vi "pattern_matching.vi"() -> ()   [LabVIEW 2014]
uses:
  <vilib>/userdefined/High Color/IMAQdx.ctl
  <vilib>/vision/Avi1.llb/AviRefnum.ctl
  <vilib>/vision/driver/NI_Vision_Acquisition_Software.lvlib
  <vilib>/vision/NI_Vision_Development_Module.lvlib
  <resource>/objmgr/imaqdx.rc
panel:
  in  "Länge der Spur":i32=50
  in  "Frames Per Second":u32=20
  in  "BayerPattern":u32(ring)=5 items=["None", "GB", "GR", "BG", "RG", "Use Hardware Value"]
  out "ValueString":string
  out "ValueBool":bool
  out "IPAddress":string
  in  "y":i32
  in  "x":i32
  in  "Pattern2 Farbe":u32(colorbox)=16711680
  in  "pattern3":bool
  in  "y 3":i32
  in  "x 3":i32
  out "Pattern 5":T1(plugin-control)
  in  "Pattern5 Farbe":u32(colorbox)=16711680
  in  "pattern5":bool
  in  "y 5":i32
  in  "x 5":i32
  in  "Pattern4 Farbe":u32(colorbox)=16711680
  in  "pattern4":bool
  in  "y 4":i32
  in  "x 4":i32
  out "Pattern 4":T1(plugin-control)
  in  "Template File Path (Pattern Matching 4":path=path "C:/Users/Kroll/Desktop/Test_04012016/Pattern/templet_invertiert_2.png"
  in  "Template File Path (Pattern Matching 5":path=path "C:/Users/Kroll/Desktop/Test_04012016/Pattern/TEST_PAINT.png"
  in  "Pattern2 Farbe":u32(colorbox)=16711680
  in  "pattern2":bool
  out "Pattern 3":T1(plugin-control)
  in  "Template File Path (Pattern Matching 3":path=path "C:/Users/Kroll/Desktop/Test_04012016/Pattern/pattern3.png"
  out "Pattern1":T1(plugin-control)
  out "Pattern 2":T1(plugin-control)
  in  "Pattern1 Farbe":u32(colorbox)=16711680
  in  "pattern1":bool
  out "Acquired Frames/s":dbl
  in  "Länge des Pfeils":sgl=80.0
  in  "Aufnahme Starten":bool
  out "Selected Path":path
  in  "Max Data Size":u32=10000
  in  "y 2":i32
  in  "x 2":i32
  out "Processed Frames/s":dbl
  in  "Template File Path (Pattern Matching 2":path=path "C:/Users/Kroll/Desktop/Test_04012016/Pattern/pattern_test_1412.png"
  in  "millisecond multiple":u32
  in  "Mittelpunktgröße":sgl
  out "date/time string":string
  in  "file path (dialog if empty)":path=path "I:/123.txt"
  in  "Template File Path (Pattern Matching 1)":path=path "C:/Users/Kroll/Desktop/Test_04012016/Pattern/pattern_1412.png"
  in  "Parameters Pattern":T2={"Number of Matches Requested"=1, "Minimum Match Score"=800.0, "Angle Ranges"=[{"Start Angle"=-180.0, "End Angle"=180.0}, {"Start Angle"=0.0, "End Angle"=360.0}]}
  in  "Programm anhalten":bool
  out "Threshold Image 2":T1(plugin-control)
  out "Image 2":T1(plugin-control)
  # "Speicherort der Log Datei"
  # "Program Delay einstellen"
  # "Zum Rauszoomen Shift benutzen ->"
  # "Aufnahme"
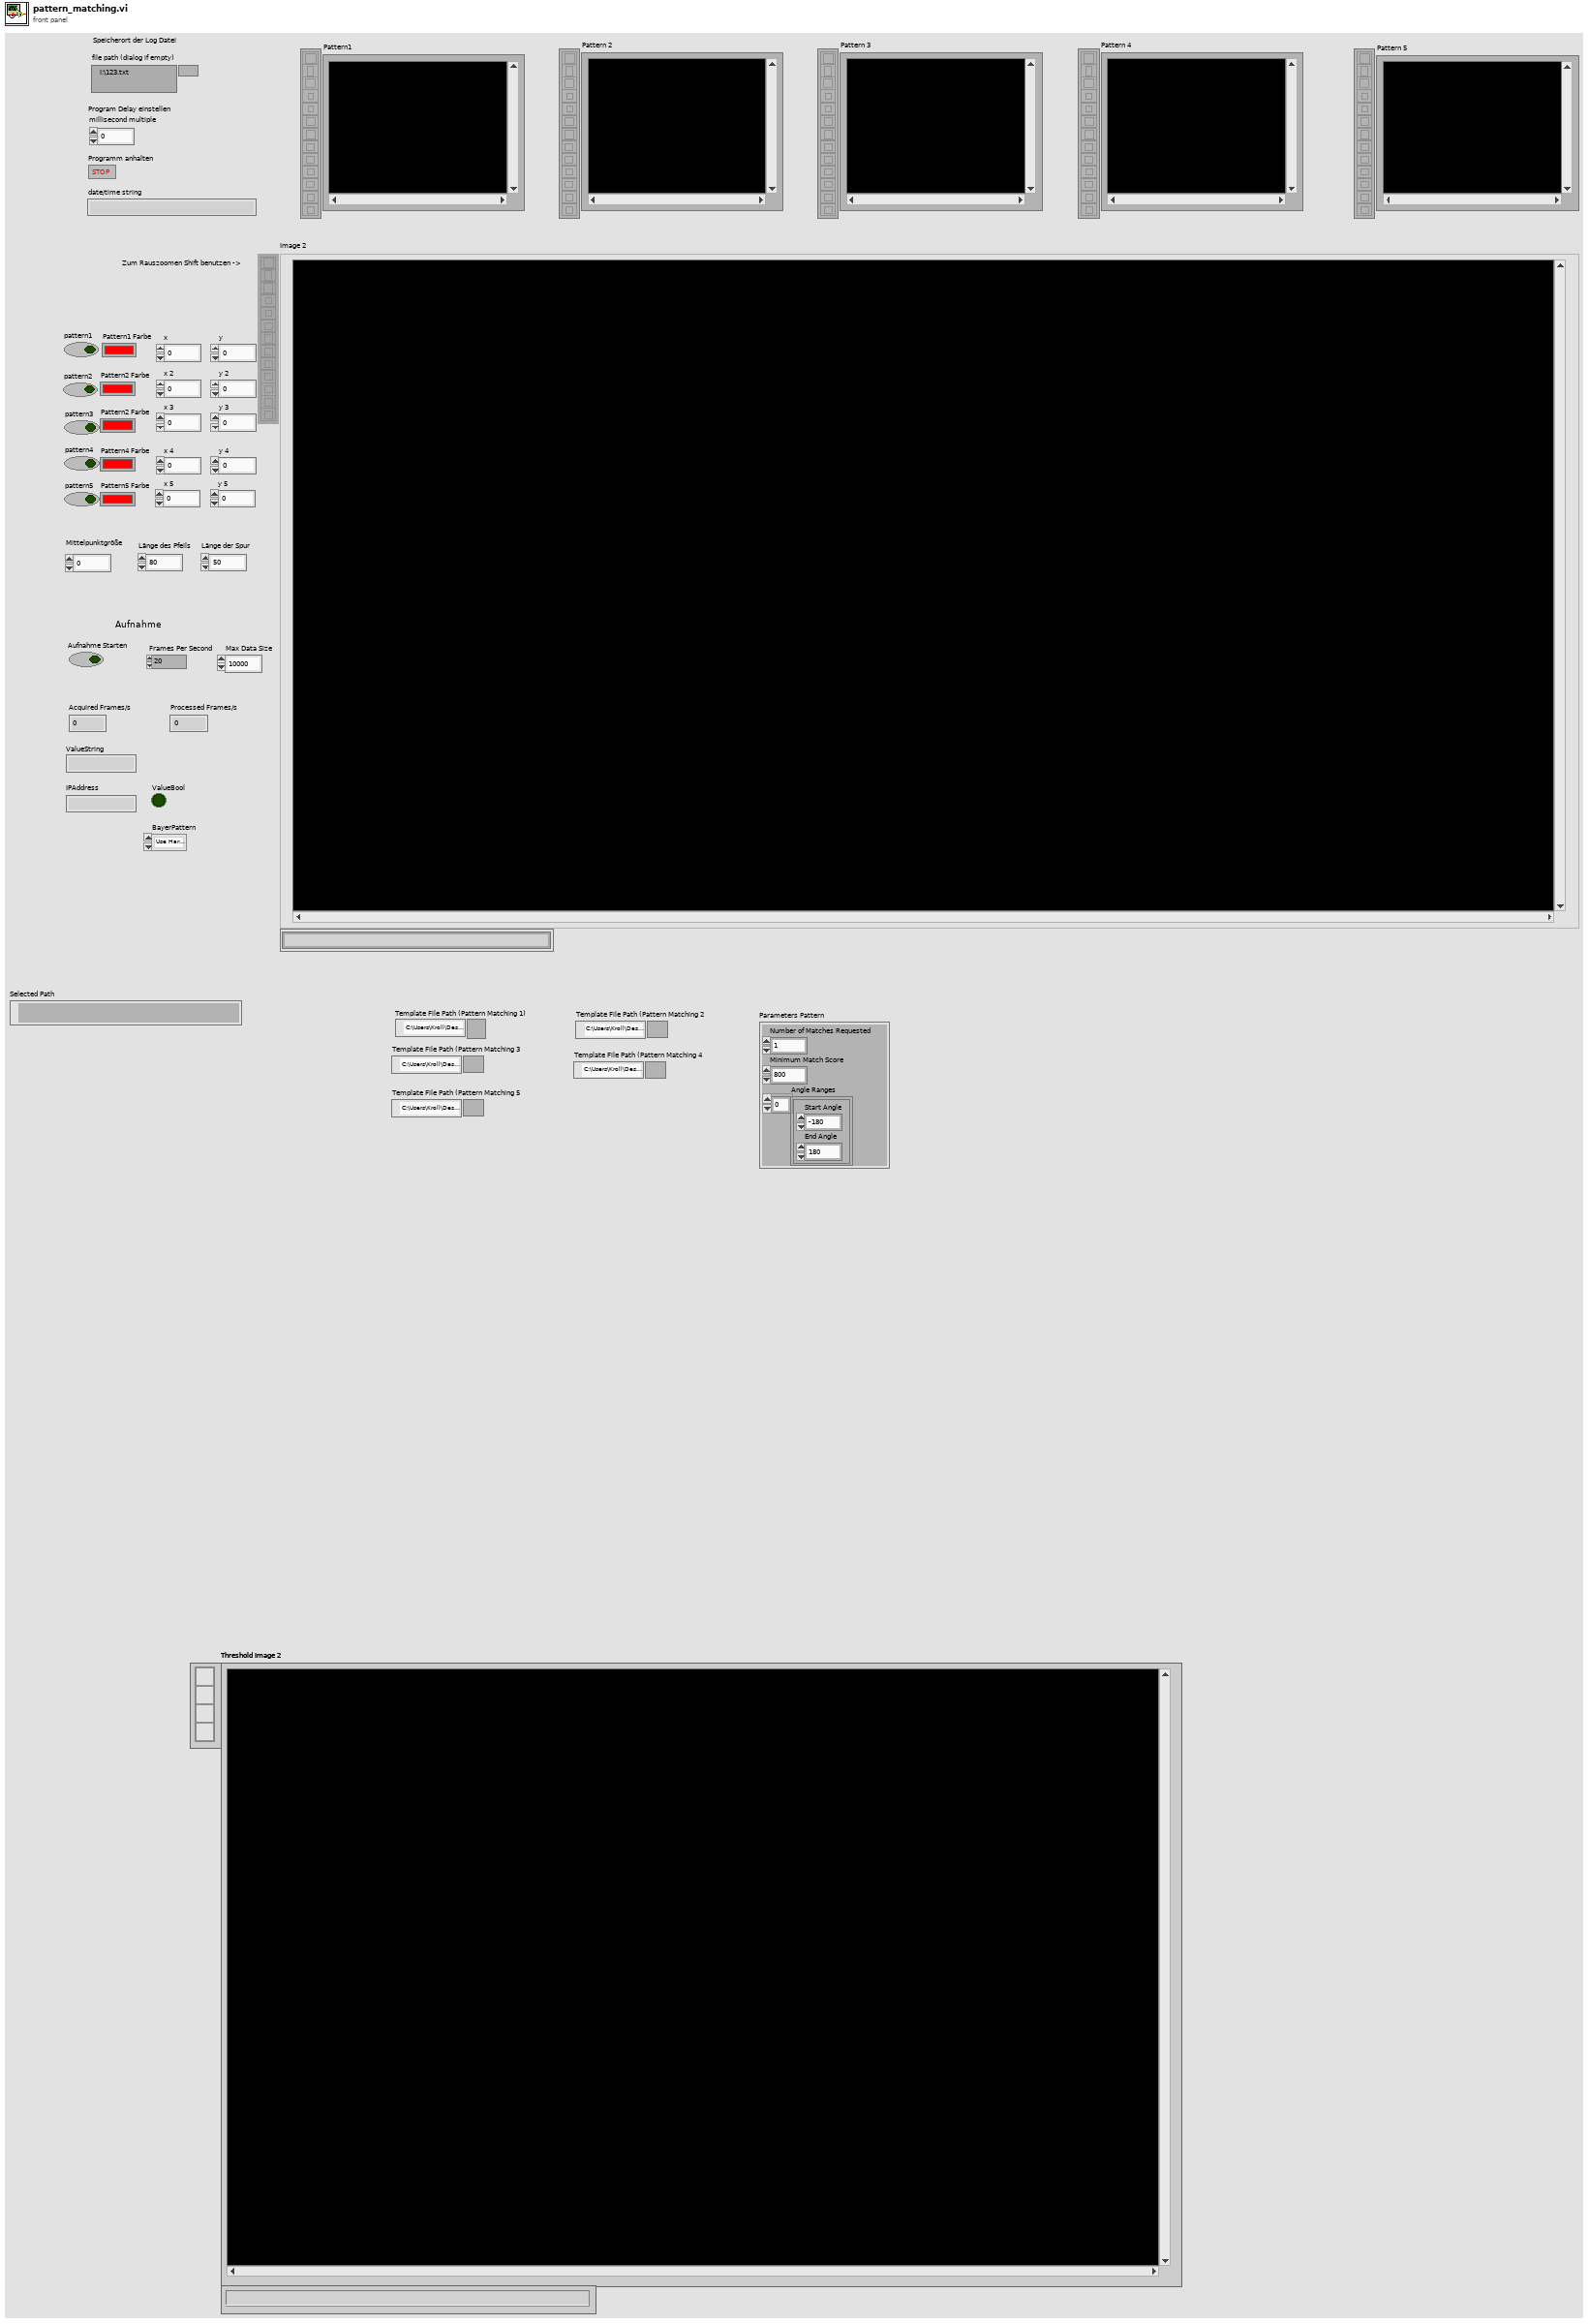
[diagram p1: front panel]
types:
  T1 = typedef "IMAQ Image.ctl" = refnum<image>
  T2 = cluster{"Number of Matches Requested":i32, "Minimum Match Score":sgl, "Angle Ranges":cluster{"Start Angle":sgl, "End Angle":sgl}[]}
  T3 = typedef "IMAQdx.ctl" = refnum<k21>
  T4 = typedef "Image Type" = u32
  T5 = enum16{"open", "replace", "create", "open or create", "replace or create", "replace or create with confirmation"}
  T6 = typedef "AviRefnum.ctl" = refnum<k1>
  T7 = enum32{"existing file", "new file", "new or existing file", "existing dir", "new dir", "new or existing dir", "existing file (use LLBs)", "new file (use LLBs)", "new or existing file (use LLBs)", "new or existing file or directory (use LLBs)"}
  T8 = cluster{"Position":cluster{"x":sgl, "y":sgl}, "Angle":sgl, "Scale":sgl, "Score":sgl, "Bounding Box":cluster{"x":sgl, "y":sgl}[]}[]
  T9 = typedef "ROI Descriptor" = cluster{"Global Rectangle":i32[], "Contours":cluster{"ID":enum32{"External", "Internal"}, "Type":u32, "Coordinates":i32[]}[]}
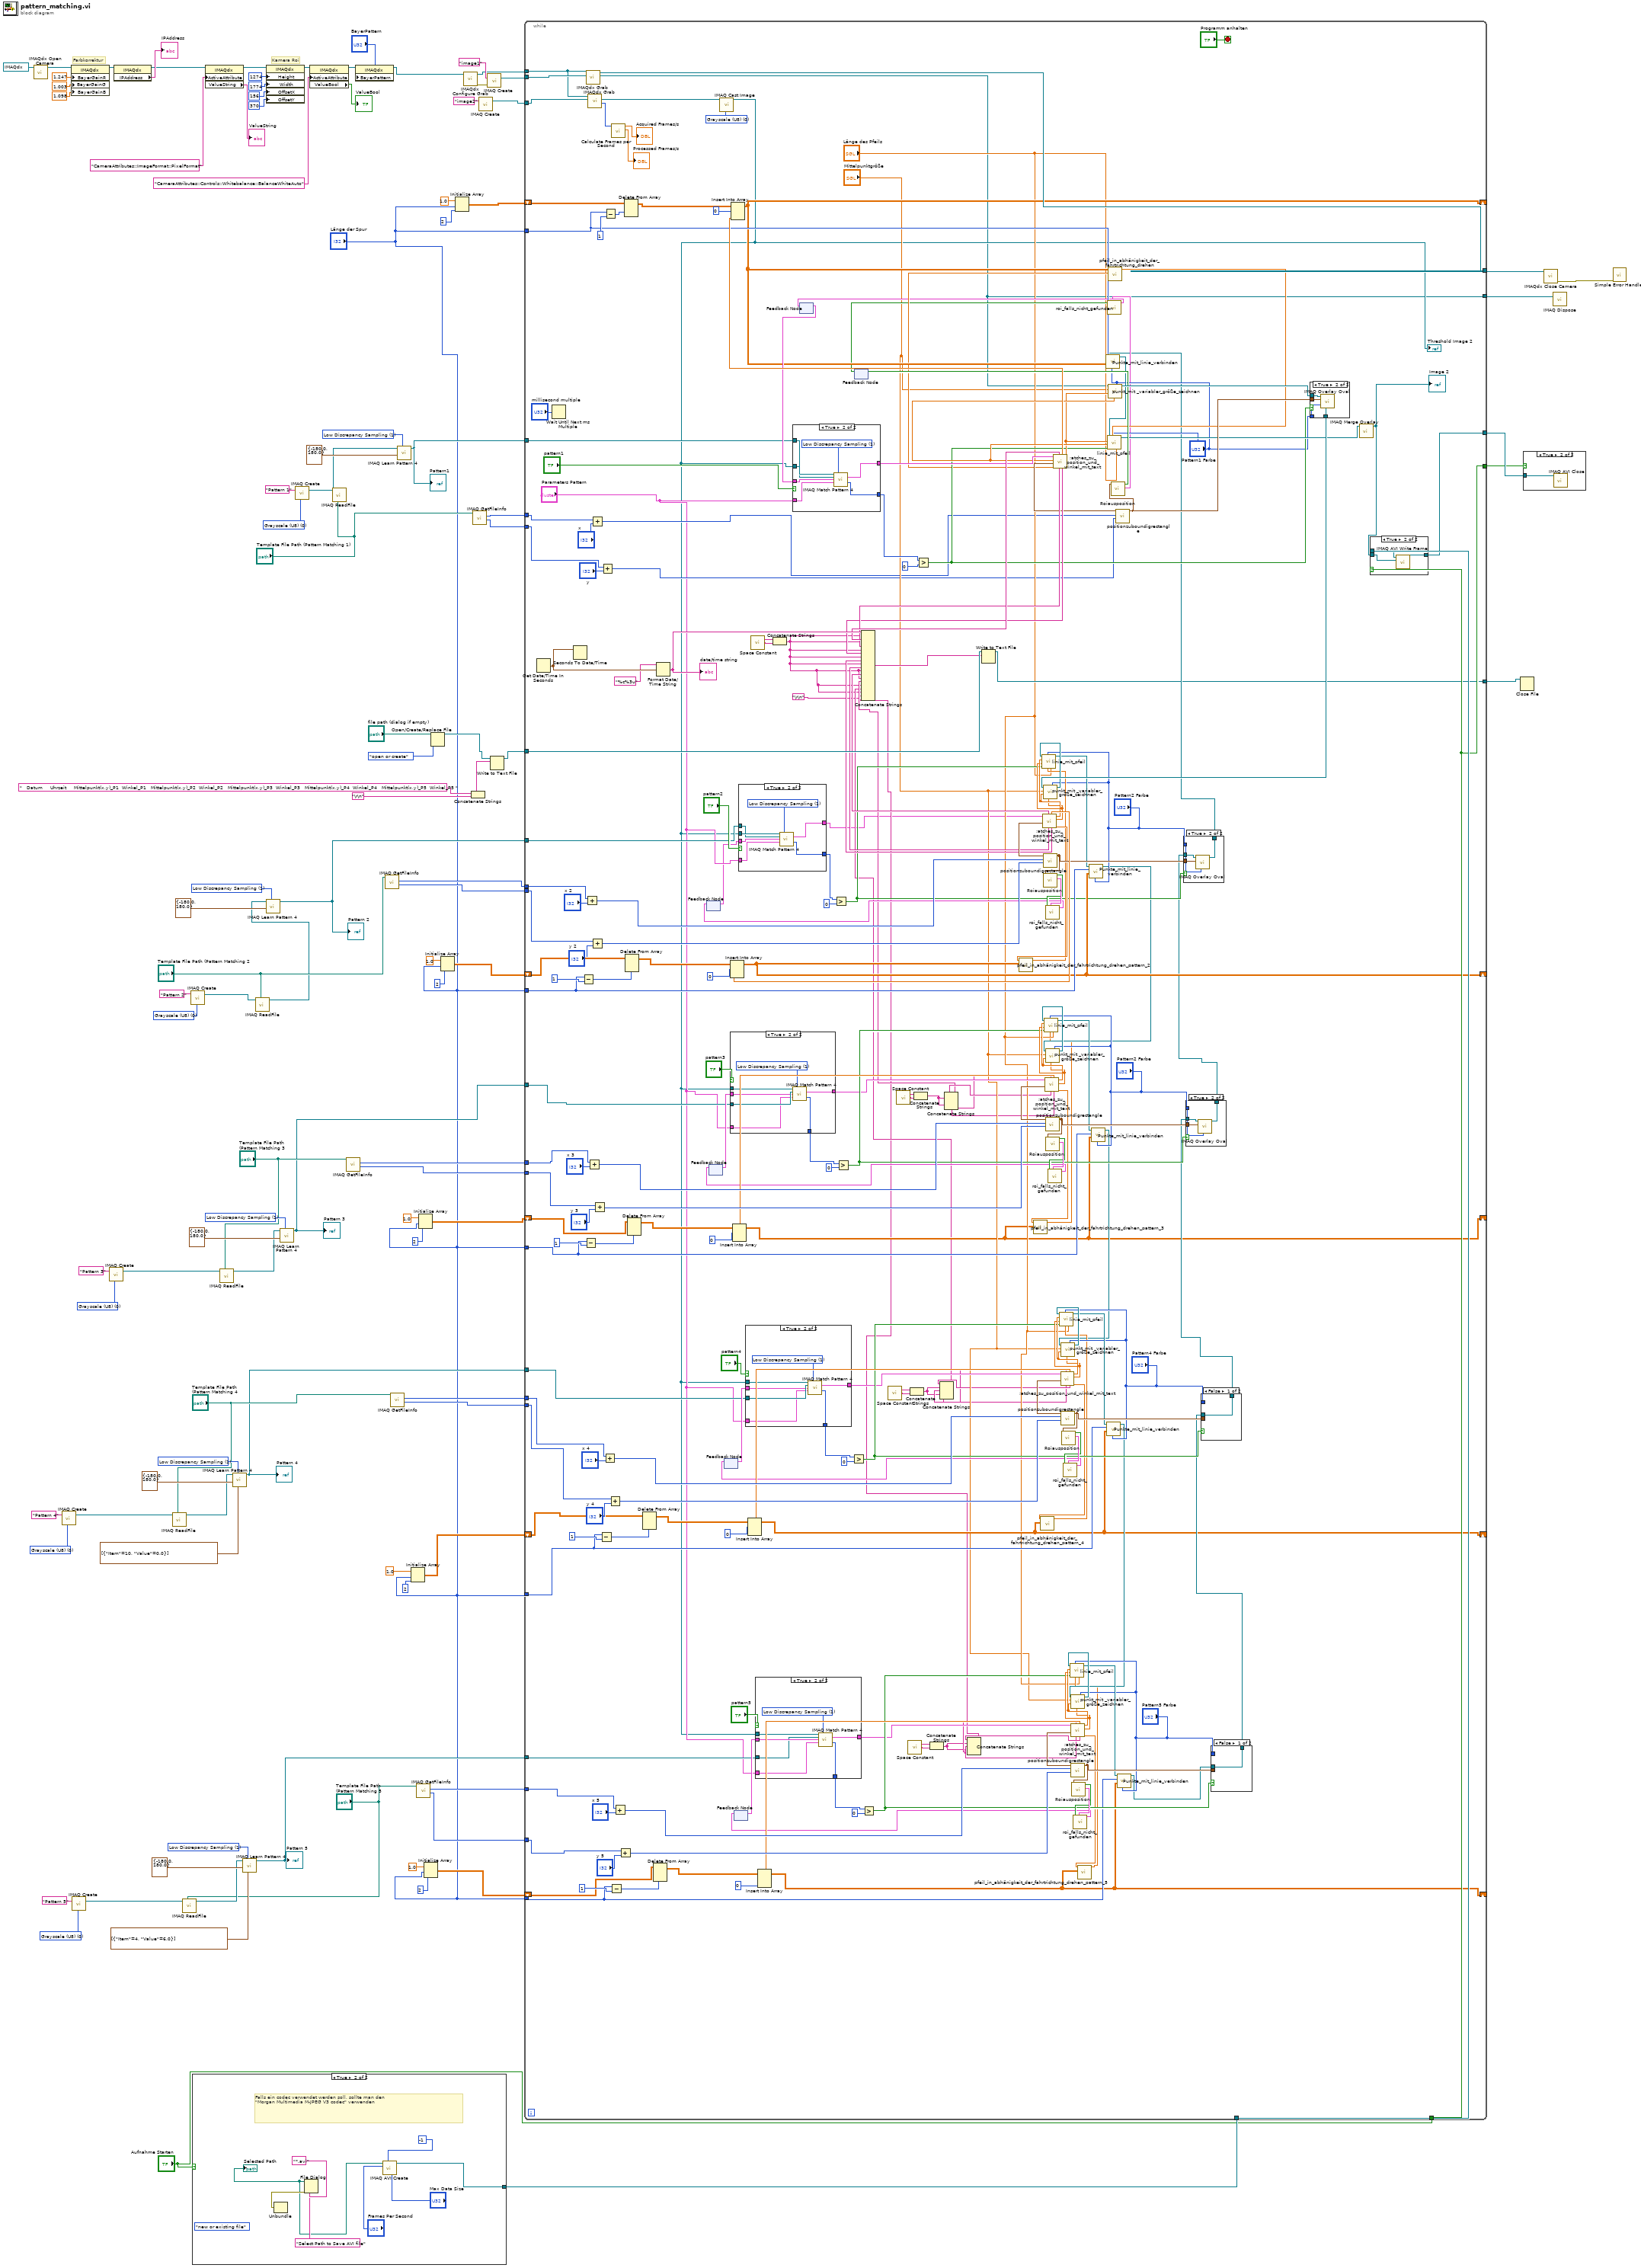
[diagram p0: block diagram]
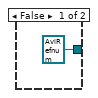
[diagram p3: hidden frame]
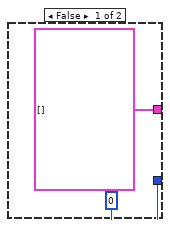
[diagram p4: hidden frame]
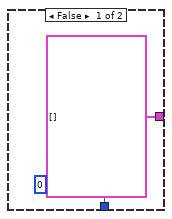
[diagram p5: hidden frame]
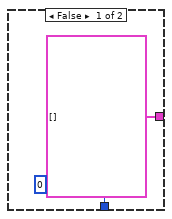
[diagram p7: hidden frame]
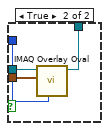
[diagram p8: hidden frame]
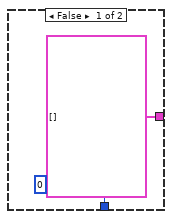
[diagram p9: hidden frame]
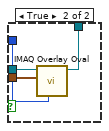
[diagram p10: hidden frame]
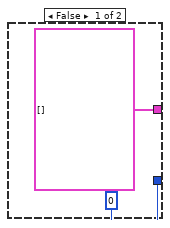
[diagram p11: hidden frame]
diagram:
  w6 = 1 items=["All", "Low Discrepancy Sampling", "Grayscale Value Pyramid", "Gradients Pyramid"] ("Algorithm")
  w32 = T4 0 items=["Grayscale (U8)", "Grayscale (I16)", "Grayscale (SGL)", "Complex (CSG)", "RGB (U32)", "HSL (U32)", "RGB (U64)", "Grayscale (U16)"] ("Image Type")
  w36 = 1 items=["All", "Low Discrepancy Sampling", "Grayscale Value Pyramid", "Gradients Pyramid"] ("Algorithm")
  w41 = T4 0 items=["Grayscale (U8)", "Grayscale (I16)", "Grayscale (SGL)", "Complex (CSG)", "RGB (U32)", "HSL (U32)", "RGB (U64)", "Grayscale (U16)"] ("Image Type")
  w45 = 1 items=["All", "Low Discrepancy Sampling", "Grayscale Value Pyramid", "Gradients Pyramid"] ("Algorithm")
  w59 = T4 0 items=["Grayscale (U8)", "Grayscale (I16)", "Grayscale (SGL)", "Complex (CSG)", "RGB (U32)", "HSL (U32)", "RGB (U64)", "Grayscale (U16)"] ("Image Type")
  w63 = 1 items=["All", "Low Discrepancy Sampling", "Grayscale Value Pyramid", "Gradients Pyramid"] ("Algorithm")
  w72 = T4 0 items=["Grayscale (U8)", "Grayscale (I16)", "Grayscale (SGL)", "Complex (CSG)", "RGB (U32)", "HSL (U32)", "RGB (U64)", "Grayscale (U16)"] ("Image Type")
  w76 = 1 items=["All", "Low Discrepancy Sampling", "Grayscale Value Pyramid", "Gradients Pyramid"] ("Algorithm")
  w78 = T4 0 items=["Grayscale (U8)", "Grayscale (I16)", "Grayscale (SGL)", "Complex (CSG)", "RGB (U32)", "HSL (U32)", "RGB (U64)", "Grayscale (U16)"] ("Image Type")
  # "Kamera Roi"
  # "Farbkorrektur"
  n1 = call <vilib>:"IMAQdx Open Camera.vi"("Session In"=T3 "cam0") -> ("Session Out"=w15:T3)  [unwired: 9 in, 1 out]
  n2 = call "IMAQ Create"("Image Name"="Pattern 4", "Image Type"=w41) -> ("New Image"=w42:T1)  [unwired: 3 in, 1 out]
  n3 = property class="IMAQdx"(reference=w15, "BayerGainR"=1.247, "BayerGainG"=1.003, "BayerGainB"=1.098) -> (reference out=w19:T3)  [unwired: 1 in, 1 out]
  n4 = call "IMAQ Create"("Image Name"="Pattern 5", "Image Type"=w32) -> ("New Image"=w33:T1)  [unwired: 3 in, 1 out]
  n5 = call "IMAQ Create"("Image Name"="Pattern 3", "Image Type"=w59) -> ("New Image"=w60:T1)  [unwired: 3 in, 1 out]
  n6 = property class="IMAQdx"(reference=w19) -> (reference out=w1:T3, "IPAddress"=→"IPAddress":string)  [unwired: 1 in, 1 out]
  n7 = call "IMAQ ReadFile"("File Path"="Template File Path (Pattern Matching 4", "Image"=w42) -> ("Image Out"=w40:T1)  [unwired: 5 in, 4 out]
  n8 = call "IMAQ ReadFile"("File Path"="Template File Path (Pattern Matching 5", "Image"=w33) -> ("Image Out"=w31:T1)  [unwired: 5 in, 4 out]
  n9 = call "IMAQ Create"("Image Name"="Pattern 2", "Image Type"=w78) -> ("New Image"=w79:T1)  [unwired: 3 in, 1 out]
  n10 = case shown="True" "Aufnahme Starten" {
    tunnel: [T6 refnum ("Avi Refnum") w113] -> w84
    frame False {
    }
    frame True {
      (unwired) T7."new or existing file" ("select mode (2)")
      # "Falls ein codec verwendet werden soll, sollte man den \n\"Morgan Multimedia M-JPEG V3 codec\" verwenden"
      n11 = File Dialog(6:"*.avi" ("pattern"), 7:"Select Path to Save AVI file" ("prompt")) -> (0:w116:errorcluster, 3:w115:path)  [unwired: 1 in, 6 out]
      "Selected Path" <- w115
      n12 = Unbundle(w116) -> ()  [unwired: 3 out]
      n13 = call "IMAQ AVI Create"("Max Data Size"="Max Data Size", "quality"=-1, "Frames Per Second"="Frames Per Second", "AVI Path"=w115) -> ("Avi Refnum"=w113:T6)  [unwired: 6 in, 1 out]
    }
  }
  n14 = property class="IMAQdx"(reference=w1, "ActiveAttribute"="CameraAttributes::ImageFormat::PixelFormat") -> (reference out=w11:T3, "ValueString"=→"ValueString":string)  [unwired: 1 in, 1 out]
  n15 = call "IMAQ ReadFile"("File Path"="Template File Path (Pattern Matching 3", "Image"=w60) -> ("Image Out"=w58:T1)  [unwired: 5 in, 4 out]
  n16 = call "IMAQ Learn Pattern 4"("Advanced Options"=cluster{"Item":u16, "Value":dbl}[] [{"Item"=10, "Value"=0.0}], "Algorithm"=w45, "Angle Range"=cluster{"Start Angle":sgl, "End Angle":sgl} {"Start Angle"=-180.0, "End Angle"=180.0}, "Image"=w40) -> ("Template Image Out"=w37:T1)  [unwired: 5 in, 2 out]
  "Pattern 4" <- w37
  n17 = call "IMAQ Learn Pattern 4"("Advanced Options"=cluster{"Item":u16, "Value":dbl}[] [{"Item"=4, "Value"=6.0}], "Algorithm"=w36, "Angle Range"=cluster{"Start Angle":sgl, "End Angle":sgl} {"Start Angle"=-180.0, "End Angle"=180.0}, "Image"=w31) -> ("Template Image Out"=w28:T1)  [unwired: 5 in, 2 out]
  "Pattern 5" <- w28
  n18 = call "IMAQ ReadFile"("File Path"="Template File Path (Pattern Matching 2", "Image"=w79) -> ("Image Out"=w4:T1)  [unwired: 5 in, 4 out]
  n19 = call "IMAQ Learn Pattern 4"("Algorithm"=w6, "Angle Range"=cluster{"Start Angle":sgl, "End Angle":sgl} {"Start Angle"=-180.0, "End Angle"=180.0}, "Image"=w4) -> ("Template Image Out"=w3:T1)  [unwired: 6 in, 2 out]
  "Pattern 2" <- w3
  n20 = property class="IMAQdx"(reference=w11, "Height"=u32 1274, "Width"=u32 1774, "OffsetX"=u32 156, "OffsetY"=u32 370) -> (reference out=w12:T3)  [unwired: 1 in, 1 out]
  n21 = call "IMAQ Learn Pattern 4"("Algorithm"=w63, "Angle Range"=cluster{"Start Angle":sgl, "End Angle":sgl} {"Start Angle"=-180.0, "End Angle"=180.0}, "Image"=w58) -> ("Template Image Out"=w56:T1)  [unwired: 6 in, 2 out]
  "Pattern 3" <- w56
  n22 = call "IMAQ Create"("Image Name"="Pattern 1", "Image Type"=w72) -> ("New Image"=w73:T1)  [unwired: 3 in, 1 out]
  n23 = property class="IMAQdx"(reference=w12, "ActiveAttribute"="CameraAttributes::Controls::Whitebalance::BalanceWhiteAuto") -> (reference out=w23:T3, "ValueBool"=→"ValueBool":bool)  [unwired: 1 in, 1 out]
  n24 = call "IMAQ ReadFile"("File Path"="Template File Path (Pattern Matching 1)", "Image"=w73) -> ("Image Out"=w70:T1)  [unwired: 5 in, 4 out]
  n25 = call "IMAQ GetFileInfo"("File Path"="Template File Path (Pattern Matching 3") -> ("Y Resolution"=w64:i32, "X Resolution"=w65:i32)  [unwired: 4 in, 5 out]
  n26 = property class="IMAQdx"(reference=w23, "BayerPattern"="BayerPattern") -> (reference out=w13:T3)  [unwired: 1 in, 1 out]
  n27 = call "IMAQ GetFileInfo"("File Path"="Template File Path (Pattern Matching 2") -> ("Y Resolution"=w89:i32, "X Resolution"=w90:i32)  [unwired: 4 in, 5 out]
  n28 = call "IMAQ GetFileInfo"("File Path"="Template File Path (Pattern Matching 4") -> ("Y Resolution"=w51:i32, "X Resolution"=w52:i32)  [unwired: 4 in, 5 out]
  n29 = call "IMAQ Learn Pattern 4"("Algorithm"=w76, "Angle Range"=cluster{"Start Angle":sgl, "End Angle":sgl} {"Start Angle"=-180.0, "End Angle"=180.0}, "Image"=w70) -> ("Template Image Out"=w69:T1)  [unwired: 6 in, 2 out]
  "Pattern1" <- w69
  n30 = Initialize Array "Initialize Array"(1.0 ("element"), "Länge der Spur", 2 ("dimension size")) -> (w53:dbl[][])
  n31 = call "IMAQ GetFileInfo"("File Path"="Template File Path (Pattern Matching 5") -> ("Y Resolution"=w46:i32, "X Resolution"=w47:i32)  [unwired: 4 in, 5 out]
  n32 = Initialize Array "Initialize Array"(1.0 ("element"), "Länge der Spur", 2 ("dimension size")) -> (w66:dbl[][])
  n33 = Initialize Array "Initialize Array"(1.0 ("element"), "Länge der Spur", 2 ("dimension size")) -> (w48:dbl[][])
  n34 = Open/Create/Replace File(file path (use dialog)="file path (dialog if empty)", operation (0:open)=T5."open or create") -> (refnum out=w97:refnum<file>)  [unwired: 4 in, 2 out]
  n35 = Initialize Array "Initialize Array"(1.0 ("element"), "Länge der Spur", 2 ("dimension size")) -> (w86:dbl[][])
  n36 = Initialize Array "Initialize Array"(1.0 ("element"), "Länge der Spur", 2 ("dimension size")) -> (w92:dbl[][])
  n37 = call <vilib>:"IMAQdx Configure Grab.vi"("Session In"=w13) -> ("error out"=w110:errorcluster, "Session Out"=w108:T3)  [unwired: 9 in]
  n38 = Concatenate Strings("   Datum     Uhrzeit     Mittelpunkt(x,y)_P1  Winkel_P1   Mittelpunkt(x,y)_P2  Winkel_P2   Mittelpunkt(x,y)_P3  Winkel_P3   Mittelpunkt(x,y)_P4  Winkel_P4   Mittelpunkt(x,y)_P5  Winkel_P5 " ("string"), "\r\n") -> (w94:string)
  n39 = call "IMAQ GetFileInfo"("File Path"="Template File Path (Pattern Matching 1)") -> ("Y Resolution"=w100:i32, "X Resolution"=w101:i32)  [unwired: 4 in, 5 out]
  n40 = call "IMAQ Create"("Image Name"="image2") -> ("New Image"=w103:T1)  [unwired: 4 in, 1 out]
  n41 = call "IMAQ Create"("Image Name"="image1", "error in (no error)"=w110) -> ("New Image"=w107:T1)  [unwired: 3 in, 1 out]
  n42 = Write to Text File(file (use dialog)=w97, text=w94) -> (refnum out=w96:refnum<file>)  [unwired: 2 in, 2 out]
  n43 = while {
    tunnel: w108 -> [w346]
    tunnel: w107 -> [w347]
    tunnel: [w348] -> w105
    tunnel: [w120] -> w102
    tunnel: w103 -> [w345]
    tunnel: w101 -> [w152]
    tunnel: w100 -> [w154]
    tunnel: w96 -> [w341]
    shift-right: [w279] -> _
    shift-left: w92 -> [w332]
    tunnel: "Länge der Spur" -> [w321]
    tunnel: w90 -> [w318]
    tunnel: w89 -> [w316]
    tunnel: "Länge der Spur" -> [w311]
    shift-right: [w284] -> _
    shift-left: w86 -> [w323]
    tunnel: w84 -> [w304]
    tunnel: [w303] -> w83
    tunnel: "Aufnahme Starten" -> [w295]
    tunnel: [w295] -> w81
    tunnel: w3 -> [w126]
    tunnel: w69 -> [w268]
    tunnel: "Länge der Spur" -> [w166]
    shift-right: [w158] -> _
    shift-left: w66 -> [w167]
    tunnel: w65 -> [w169]
    tunnel: w64 -> [w168]
    tunnel: w56 -> [w170]
    tunnel: "Länge der Spur" -> [w234]
    tunnel: w52 -> [w238]
    tunnel: w51 -> [w236]
    shift-right: [w197] -> _
    shift-left: w53 -> [w235]
    tunnel: "Länge der Spur" -> [w206]
    shift-right: [w201] -> _
    shift-left: w48 -> [w207]
    tunnel: w47 -> [w209]
    tunnel: w46 -> [w208]
    tunnel: w37 -> [w237]
    tunnel: w28 -> [w129]
    tunnel: [w202] -> w27
    stop <- "Programm anhalten" stop-if-true
    w274 = T4 0 items=["Grayscale (U8)", "Grayscale (I16)", "Grayscale (SGL)", "Complex (CSG)", "RGB (U32)", "HSL (U32)", "RGB (U64)", "Grayscale (U16)"] ("Image Type")
    n44 = Get Date/Time In Seconds() -> (seconds since 1Jan1904=w340:timestamp)
    n45 = Wait Until Next ms Multiple(millisecond multiple="millisecond multiple") -> ()  [unwired: 1 out]
    n46 = Seconds To Date/Time(time stamp (now)=w340) -> ()  [unwired: 1 in, 1 out]
    n47 = Subtract(x=w311, y=1) -> (x-y=w324:i32)
    n48 = Subtract(x=w166, y=1) -> (x-y=w192:i32)
    n49 = Add(x=w318, y="x 2") -> (x+y=w319:i32)
    n50 = call <vilib>:"IMAQdx Grab.vi"("Image In"=w347, "Session In"=w346) -> ("Image Out"=w120:T1, "Session Out"=w348:T3)  [unwired: 6 in, 2 out]
    n51 = Add(x=w169, y="x 3") -> (x+y=w191:i32)
    n52 = call <vilib>:"IMAQdx Grab.vi"("Image In"=w345, "Session In"=w346) -> ("Buffer Number Out"=w343:u32, "Image Out"=w121:T1)  [unwired: 6 in, 2 out]
    n53 = Add(x=w152, y="x") -> (x+y=w151:i32)
    n54 = Add(x=w316, y="y 2") -> (x+y=w314:i32)
    n55 = Add(x=w168, y="y 3") -> (x+y=w188:i32)
    n56 = Subtract(x=w234, y=1) -> (x-y=w260:i32)
    n57 = Add(x=w154, y="y") -> (x+y=w153:i32)
    n58 = Add(x=w238, y="x 4") -> (x+y=w259:i32)
    n59 = Subtract(x=w321, y=1) -> (x-y=w328:i32)
    n60 = Add(x=w236, y="y 4") -> (x+y=w256:i32)
    n61 = Subtract(x=w206, y=1) -> (x-y=w230:i32)
    n62 = call <vilib>:"Calculate Frames per Second.vi"("Buffer Number"=w343) -> ("Processed Frames/s"=→"Processed Frames/s":dbl, "Acquired Frames/s"=→"Acquired Frames/s":dbl)  [unwired: 8 in, 1 out]
    n63 = Add(x=w209, y="x 5") -> (x+y=w229:i32)
    n64 = Add(x=w208, y="y 5") -> (x+y=w226:i32)
    n65 = Delete From Array "Delete From Array"(array=w332, index (row)=w328) -> (array with subset deleted=w331:dbl[][])  [unwired: 2 in, 1 out]
    n66 = Delete From Array "Delete From Array"(array=w323, index (row)=w324) -> (array with subset deleted=w327:dbl[][])  [unwired: 2 in, 1 out]
    n67 = Delete From Array "Delete From Array"(array=w167, index (row)=w192) -> (array with subset deleted=w195:dbl[][])  [unwired: 2 in, 1 out]
    n68 = Delete From Array "Delete From Array"(array=w235, index (row)=w260) -> (array with subset deleted=w263:dbl[][])  [unwired: 2 in, 1 out]
    n69 = Delete From Array "Delete From Array"(array=w207, index (row)=w230) -> (array with subset deleted=w233:dbl[][])  [unwired: 2 in, 1 out]
    n70 = Format Date/Time String(time format string (%c)="%c%3u", seconds (now)=w340) -> (date/time string=w338:string)  [unwired: 1 in]
    "date/time string" <- w338
    n71 = feedback #1() -> (w124:T9)  [unwired: 1 in]
    n72 = feedback #2() -> (w176:T9)  [unwired: 1 in]
    n73 = call "IMAQ Cast Image"("Image Type"=w274, "Image Src"=w121) -> ("Image Dst Out"=w122:T1)  [unwired: 8 in, 1 out]
    "Threshold Image 2" <- w122
    n74 = feedback #3() -> (w244:T9)  [unwired: 1 in]
    n75 = case shown="True" "pattern3" {
      tunnel: w170 -> [_ w366]
      tunnel: w176 -> [_ w364]
      tunnel: "Parameters Pattern" -> [_ w363]
      tunnel: [0 ("Number of Matches") w362] -> w175
      tunnel: [T8 [] ("Matches (pixel)") w361] -> w174
      tunnel: w122 -> [_ w360]
      frame False {
      }
      frame True {
        w365 = 1 items=["All", "Low Discrepancy Sampling", "Grayscale Value Pyramid", "Gradients Pyramid"] ("Algorithm")
        n76 = call "IMAQ Match Pattern 4"("Image"=w360, "Algorithm"=w365, "Template Image"=w366, "ROI Descriptor"=w364, "Parameters"=w363) -> ("Matches (pixel)"=w361:T8, "Number of Matches"=w362:i32)  [unwired: 6 in, 3 out]
      }
    }
    n77 = feedback #4() -> (w130:T9)  [unwired: 1 in]
    n78 = case shown="True" "pattern2" {
      tunnel: [0 ("Number of Matches (Pattern Matching 1)") w354] -> w123
      tunnel: w126 -> [_ w351]
      tunnel: w124 -> [_ w357]
      tunnel: [T8 [] ("Matches (Pattern Matching 1)") w355] -> w128
      tunnel: "Parameters Pattern" -> [_ w356]
      tunnel: w122 -> [_ w352]
      frame False {
      }
      frame True {
        w353 = 1 items=["All", "Low Discrepancy Sampling", "Grayscale Value Pyramid", "Gradients Pyramid"] ("Algorithm")
        n79 = call "IMAQ Match Pattern 4"("Image"=w352, "Algorithm"=w353, "Template Image"=w351, "ROI Descriptor"=w357, "Parameters"=w356) -> ("Matches (pixel)"=w355:T8, "Number of Matches"=w354:i32)  [unwired: 6 in, 3 out]
      }
    }
    n80 = case shown="True" "pattern4" {
      tunnel: w237 -> [_ w394]
      tunnel: w244 -> [_ w392]
      tunnel: "Parameters Pattern" -> [_ w391]
      tunnel: [0 ("Number of Matches") w390] -> w243
      tunnel: [T8 [] ("Matches (pixel)") w389] -> w242
      tunnel: w122 -> [_ w388]
      frame False {
      }
      frame True {
        w393 = 1 items=["All", "Low Discrepancy Sampling", "Grayscale Value Pyramid", "Gradients Pyramid"] ("Algorithm")
        n81 = call "IMAQ Match Pattern 4"("Image"=w388, "Algorithm"=w393, "Template Image"=w394, "ROI Descriptor"=w392, "Parameters"=w391) -> ("Matches (pixel)"=w389:T8, "Number of Matches"=w390:i32)  [unwired: 6 in, 3 out]
      }
    }
    n82 = call <vilib>:"Space Constant.vi"() -> ("String"=w265:string)
    n83 = case shown="True" "pattern5" {
      tunnel: w130 -> [_ w379]
      tunnel: "Parameters Pattern" -> [_ w378]
      tunnel: [0 ("Number of Matches") w377] -> w214
      tunnel: [T8 [] ("Matches (pixel)") w376] -> w213
      tunnel: w129 -> [_ w375]
      tunnel: w122 -> [_ w374]
      frame False {
      }
      frame True {
        w380 = 1 items=["All", "Low Discrepancy Sampling", "Grayscale Value Pyramid", "Gradients Pyramid"] ("Algorithm")
        n84 = call "IMAQ Match Pattern 4"("Image"=w374, "Algorithm"=w380, "Template Image"=w375, "ROI Descriptor"=w379, "Parameters"=w378) -> ("Matches (pixel)"=w376:T8, "Number of Matches"=w377:i32)  [unwired: 6 in, 3 out]
      }
    }
    n85 = Concatenate Strings(w265, w265) -> (w133:string)
    n86 = feedback #5() -> (w300:T9)  [unwired: 1 in]
    n87 = case shown="True" "pattern1" {
      tunnel: [0 ("Number of Matches (Pattern Matching 1)") w403] -> w277
      tunnel: w122 -> [_ w408]
      tunnel: w300 -> [_ w406]
      tunnel: [T8 [] ("Matches (Pattern Matching 1)") w404] -> w293
      tunnel: "Parameters Pattern" -> [_ w405]
      tunnel: w268 -> [_ w407]
      frame False {
      }
      frame True {
        w402 = 1 items=["All", "Low Discrepancy Sampling", "Grayscale Value Pyramid", "Gradients Pyramid"] ("Algorithm")
        n88 = call "IMAQ Match Pattern 4"("Image"=w408, "Algorithm"=w402, "Template Image"=w407, "ROI Descriptor"=w406, "Parameters"=w405) -> ("Matches (pixel)"=w404:T8, "Number of Matches"=w403:i32)  [unwired: 6 in, 3 out]
      }
    }
    n89 = Greater?(x=w123, y=0) -> (0:w275:bool)
    n90 = Greater?(x=w175, y=0) -> (0:w177:bool)
    n91 = Greater?(x=w243, y=0) -> (0:w245:bool)
    n92 = feedback #6() -> (w271:bool)  [unwired: 1 in]
    n93 = Greater?(x=w214, y=0) -> (0:w215:bool)
    n94 = call <vilib>:"Space Constant.vi"() -> ("String"=w146:string)
    n95 = call <vilib>:"Space Constant.vi"() -> ("String"=w147:string)
    n96 = call <vilib>:"Space Constant.vi"() -> ("String"=w141:string)
    n97 = Concatenate Strings(w146, w146) -> (w142:string)
    n98 = Concatenate Strings(w147, w147) -> (w136:string)
    n99 = Greater?(x=w277, y=0) -> (0:w276:bool)
    n100 = Concatenate Strings(w141, w141) -> (w137:string)
    n101 = call ";atches_zu_position_und_winkel_mit_text.vi"("Matches (Pattern Matching 1)"=w128) -> ("Angle"=w281:sgl, "Position"=w309:cluster{"x":sgl, "y":sgl}, "x"=w289:sgl, "y"=w290:sgl, "String"=w306:string, "Array"=w310:sgl[], "String 2"=w307:string, "String 3"=w308:string)  [unwired: 3 in]
    n102 = Insert Into Array "Insert Into Array"(array=w327, index (row)=0 ("index"), new element=w310) -> (w284:dbl[][])  [unwired: 1 in]
    n103 = call "pfeil_in_abhänigkeit_der_fahrtrichtung_drehen_pattern_2.vi"("Array"=w284, "Angle in"=w281) -> ("Angle out"=w280:sgl)  [unwired: 9 in]
    n104 = call "positionzuboundigrectangle.vi"("Y Resolution"=w314, "X Resolution"=w319, "Position"=w309) -> ("Cluster"=w299:cluster{dbl, dbl, dbl, dbl})  [unwired: 8 in]
    n105 = call "Roiausposition.vi"("Cluster"=w299) -> ("ROI Descriptor"=w298:T9, "Boolean"=w297:bool)  [unwired: 9 in]
    n106 = call ";atches_zu_position_und_winkel_mit_text.vi"("Matches (Pattern Matching 1)"=w174) -> ("Angle"=w159:sgl, "Position"=w185:cluster{"x":sgl, "y":sgl}, "x"=w178:sgl, "y"=w179:sgl, "String"=w150:string, "Array"=w186:sgl[], "String 2"=w149:string, "String 3"=w148:string)  [unwired: 3 in]
    n107 = Insert Into Array "Insert Into Array"(array=w195, index (row)=0 ("index"), new element=w186) -> (w158:dbl[][])  [unwired: 1 in]
    n108 = Concatenate Strings(w150, w136, w149, w136, w148) -> (w135:string)
    n109 = call "pfeil_in_abhänigkeit_der_fahrtrichtung_drehen_pattern_3.vi"("Array"=w158, "Angle in"=w159) -> ("Angle out"=w157:sgl)  [unwired: 9 in]
    n110 = call "roi_falls_nicht_gefunden.vi"("ROI Descriptor in"=w298, "Boolean"=w297) -> ("ROI Descriptor out"=w296:T9)  [unwired: 9 in]
    n111 = feedback-in #1(w296) -> ()
    n112 = call "positionzuboundigrectangle.vi"("Y Resolution"=w188, "X Resolution"=w191, "Position"=w185) -> ("Cluster"=w184:cluster{dbl, dbl, dbl, dbl})  [unwired: 8 in]
    n113 = call "Roiausposition.vi"("Cluster"=w184) -> ("ROI Descriptor"=w183:T9, "Boolean"=w182:bool)  [unwired: 9 in]
    n114 = call "roi_falls_nicht_gefunden.vi"("ROI Descriptor in"=w183, "Boolean"=w182) -> ("ROI Descriptor out"=w181:T9)  [unwired: 9 in]
    n115 = feedback-in #2(w181) -> ()
    n116 = call ";atches_zu_position_und_winkel_mit_text.vi"("Matches (Pattern Matching 1)"=w293) -> ("Angle"=w273:sgl, "Position"=w302:cluster{"x":sgl, "y":sgl}, "x"=w286:sgl, "y"=w285:sgl, "String"=w334:string, "Array"=w322:sgl[], "String 2"=w335:string, "String 3"=w336:string)  [unwired: 3 in]
    n117 = Insert Into Array "Insert Into Array"(array=w331, index (row)=0 ("index"), new element=w322) -> (w279:dbl[][])  [unwired: 1 in]
    n118 = call ";atches_zu_position_und_winkel_mit_text.vi"("Matches (Pattern Matching 1)"=w242) -> ("Angle"=w198:sgl, "Position"=w253:cluster{"x":sgl, "y":sgl}, "x"=w246:sgl, "y"=w247:sgl, "String"=w145:string, "Array"=w254:sgl[], "String 2"=w144:string, "String 3"=w143:string)  [unwired: 3 in]
    n119 = Insert Into Array "Insert Into Array"(array=w263, index (row)=0 ("index"), new element=w254) -> (w197:dbl[][])  [unwired: 1 in]
    n120 = Concatenate Strings(w145, w142, w144, w142, w143) -> (w134:string)
    n121 = call "pfeil_in_abhänigkeit_der_fahrtrichtung_drehen_pattern_4.vi"("Array"=w197, "Angle in"=w198) -> ("Angle out"=w196:sgl)  [unwired: 9 in]
    n122 = call "positionzuboundigrectangle.vi"("Y Resolution"=w256, "X Resolution"=w259, "Position"=w253) -> ("Cluster"=w252:cluster{dbl, dbl, dbl, dbl})  [unwired: 8 in]
    n123 = call "Roiausposition.vi"("Cluster"=w252) -> ("ROI Descriptor"=w251:T9, "Boolean"=w250:bool)  [unwired: 9 in]
    n124 = call "roi_falls_nicht_gefunden.vi"("ROI Descriptor in"=w251, "Boolean"=w250) -> ("ROI Descriptor out"=w249:T9)  [unwired: 9 in]
    n125 = feedback-in #3(w249) -> ()
    n126 = call ";atches_zu_position_und_winkel_mit_text.vi"("Matches (Pattern Matching 1)"=w213) -> ("Angle"=w199:sgl, "Position"=w223:cluster{"x":sgl, "y":sgl}, "x"=w216:sgl, "y"=w217:sgl, "String"=w140:string, "Array"=w224:sgl[], "String 2"=w139:string, "String 3"=w138:string)  [unwired: 3 in]
    n127 = Insert Into Array "Insert Into Array"(array=w233, index (row)=0 ("index"), new element=w224) -> (w201:dbl[][])  [unwired: 1 in]
    n128 = Concatenate Strings(w140, w137, w139, w137, w138) -> (w132:string)
    n129 = Concatenate Strings(w338, w133, w336, w133, w335, w133, w334, w133, w306, w133, w307, w133, w308, w133, w135, w133, w134, w133, w132, "\r\n") -> (w337:string)
    n130 = Write to Text File(file (use dialog)=w341, text=w337) -> (refnum out=w202:refnum<file>)  [unwired: 2 in, 2 out]
    n131 = call "positionzuboundigrectangle.vi"("Y Resolution"=w226, "X Resolution"=w229, "Position"=w223) -> ("Cluster"=w222:cluster{dbl, dbl, dbl, dbl})  [unwired: 8 in]
    n132 = call "Roiausposition.vi"("Cluster"=w222) -> ("ROI Descriptor"=w221:T9, "Boolean"=w220:bool)  [unwired: 9 in]
    n133 = call "roi_falls_nicht_gefunden.vi"("ROI Descriptor in"=w221, "Boolean"=w220) -> ("ROI Descriptor out"=w219:T9)  [unwired: 9 in]
    n134 = feedback-in #4(w219) -> ()
    n135 = call "pfeil_in_abhänigkeit_der_fahrtrichtung_drehen_pattern_5.vi"("Array"=w201, "Angle in"=w199) -> ("Angle out"=w200:sgl)  [unwired: 9 in]
    n136 = call "pfeil_in_abhänigkeit_der_fahrtrichtung_drehen.vi"("Angle in"=w273, "Array"=w279) -> ("Angle out"=w278:sgl)  [unwired: 9 in]
    n137 = call "punkt_mit _variabler_größe_zeichnen.vi"("Color"="Pattern1 Farbe", "x"=w286, "y"=w285, "größe"="Mittelpunktgröße", "Refnum in"=w120) -> ("Refnum out"=w320:T1)  [unwired: 5 in, 1 out]
    n138 = call "positionzuboundigrectangle.vi"("Y Resolution"=w153, "X Resolution"=w151, "Position"=w302) -> ("Cluster"=w294:cluster{dbl, dbl, dbl, dbl})  [unwired: 8 in]
    n139 = call "Roiausposition.vi"("Cluster"=w294) -> ("ROI Descriptor"=w269:T9, "Boolean"=w301:bool)  [unwired: 9 in]
    n140 = feedback-in #6(w301) -> ()
    n141 = call "roi_falls_nicht_gefunden.vi"("ROI Descriptor in"=w269, "Boolean"=w271) -> ("ROI Descriptor out"=w270:T9)  [unwired: 9 in]
    n142 = feedback-in #5(w270) -> ()
    n143 = case shown="True" w276 {
      tunnel: w294 -> [_ w422]
      tunnel: [w418 w421] -> w292
      tunnel: w320 -> [w418 w420]
      tunnel: "Pattern1 Farbe" -> [_ w419]
      frame False {
      }
      frame True {
        n144 = call "IMAQ Overlay Oval"("Color"=w419, "Bounding Rectangle"=w422, "Image"=w420) -> ("Image Out"=w421:T1)  [unwired: 7 in, 1 out]
      }
    }
    n145 = call "punkt_mit _variabler_größe_zeichnen.vi"("Color"="Pattern2 Farbe", "x"=w289, "y"=w290, "größe"="Mittelpunktgröße", "Refnum in"=w292) -> ("Refnum out"=w291:T1)  [unwired: 5 in, 1 out]
    n146 = call "linie_mit_pfeil.vi"("Richtungspfeillänge"="Länge des Pfeils", "Angle"=w280, "Color"="Pattern2 Farbe", "Boolean"=w275, "x"=w289, "y"=w290, "Refnum in"=w291) -> ("Refnum out"=w267:T1)  [unwired: 4 in]
    n147 = call "Punkte_mit_linie_verbinden.vi"("Color"="Pattern2 Farbe", "Array"=w284, "dimension size"=w311, "Refnum in"=w267) -> ("Refnum out"=w163:T1)  [unwired: 7 in]
    n148 = call "punkt_mit _variabler_größe_zeichnen.vi"("Color"="Pattern2 Farbe", "x"=w178, "y"=w179, "größe"="Mittelpunktgröße", "Refnum in"=w163) -> ("Refnum out"=w180:T1)  [unwired: 5 in, 1 out]
    n149 = call "linie_mit_pfeil.vi"("Richtungspfeillänge"="Länge des Pfeils", "Angle"=w157, "Color"="Pattern2 Farbe", "Boolean"=w177, "x"=w178, "y"=w179, "Refnum in"=w180) -> ("Refnum out"=w173:T1)  [unwired: 4 in]
    n150 = call "Punkte_mit_linie_verbinden.vi"("Color"="Pattern2 Farbe", "Array"=w158, "dimension size"=w166, "Refnum in"=w173) -> ("Refnum out"=w164:T1)  [unwired: 7 in]
    n151 = call "punkt_mit _variabler_größe_zeichnen.vi"("Color"="Pattern4 Farbe", "x"=w246, "y"=w247, "größe"="Mittelpunktgröße", "Refnum in"=w164) -> ("Refnum out"=w248:T1)  [unwired: 5 in, 1 out]
    n152 = call "linie_mit_pfeil.vi"("Richtungspfeillänge"="Länge des Pfeils", "Angle"=w196, "Color"="Pattern4 Farbe", "Boolean"=w245, "x"=w246, "y"=w247, "Refnum in"=w248) -> ("Refnum out"=w241:T1)  [unwired: 4 in]
    n153 = call "Punkte_mit_linie_verbinden.vi"("Color"="Pattern4 Farbe", "Array"=w197, "dimension size"=w234, "Refnum in"=w241) -> ("Refnum out"=w205:T1)  [unwired: 7 in]
    n154 = call "punkt_mit _variabler_größe_zeichnen.vi"("Color"="Pattern5 Farbe", "x"=w216, "y"=w217, "größe"="Mittelpunktgröße", "Refnum in"=w205) -> ("Refnum out"=w218:T1)  [unwired: 5 in, 1 out]
    n155 = call "linie_mit_pfeil.vi"("Richtungspfeillänge"="Länge des Pfeils", "Angle"=w200, "Color"="Pattern5 Farbe", "Boolean"=w215, "x"=w216, "y"=w217, "Refnum in"=w218) -> ("Refnum out"=w212:T1)  [unwired: 4 in]
    n156 = call "Punkte_mit_linie_verbinden.vi"("Color"="Pattern5 Farbe", "Array"=w201, "dimension size"=w206, "Refnum in"=w212) -> ("Refnum out"=w203:T1)  [unwired: 7 in]
    n157 = case shown="False" w215 {
      tunnel: w222 -> [_ w385]
      tunnel: w203 -> [w381 w384]
      tunnel: [w381 w383] -> w204
      tunnel: "Pattern5 Farbe" -> [_ w382]
      frame False {
      }
      frame True {
        n158 = call "IMAQ Overlay Oval"("Color"=w382, "Bounding Rectangle"=w385, "Image"=w384) -> ("Image Out"=w383:T1)  [unwired: 7 in, 1 out]
      }
    }
    n159 = case shown="False" w245 {
      tunnel: w252 -> [_ w399]
      tunnel: w204 -> [w395 w398]
      tunnel: [w395 w397] -> w162
      tunnel: "Pattern4 Farbe" -> [_ w396]
      frame False {
      }
      frame True {
        n160 = call "IMAQ Overlay Oval"("Color"=w396, "Bounding Rectangle"=w399, "Image"=w398) -> ("Image Out"=w397:T1)  [unwired: 7 in, 1 out]
      }
    }
    n161 = case shown="True" w177 {
      tunnel: w184 -> [_ w371]
      tunnel: [w367 w370] -> w165
      tunnel: "Pattern2 Farbe" -> [_ w369]
      tunnel: w162 -> [w367 w368]
      frame False {
      }
      frame True {
        n162 = call "IMAQ Overlay Oval"("Color"=w369, "Bounding Rectangle"=w371, "Image"=w368) -> ("Image Out"=w370:T1)  [unwired: 7 in, 1 out]
      }
    }
    n163 = case shown="True" w275 {
      tunnel: w299 -> [_ w417]
      tunnel: [w413 w416] -> w264
      tunnel: "Pattern2 Farbe" -> [_ w415]
      tunnel: w165 -> [w413 w414]
      frame False {
      }
      frame True {
        n164 = call "IMAQ Overlay Oval"("Color"=w415, "Bounding Rectangle"=w417, "Image"=w414) -> ("Image Out"=w416:T1)  [unwired: 7 in, 1 out]
      }
    }
    n165 = call "Punkte_mit_linie_verbinden.vi"("Color"="Pattern1 Farbe", "Array"=w279, "dimension size"=w321, "Refnum in"=w264) -> ("Refnum out"=w288:T1)  [unwired: 7 in]
    n166 = call "linie_mit_pfeil.vi"("Richtungspfeillänge"="Länge des Pfeils", "Angle"=w278, "Color"="Pattern1 Farbe", "Boolean"=w276, "x"=w286, "y"=w285, "Refnum in"=w288) -> ("Refnum out"=w287:T1)  [unwired: 4 in]
    n167 = call "IMAQ Merge Overlay"("Image Src"=w287) -> ("Image Dst Out"=w305:T1)  [unwired: 9 in, 1 out]
    "Image 2" <- w305
    n168 = case shown="True" w295 {
      tunnel: w305 -> [_ w412]
      tunnel: w304 -> [w409 w411]
      tunnel: [w409 w410] -> w303
      frame False {
      }
      frame True {
        n169 = call "IMAQ AVI Write Frame"("Image"=w412, "Avi Refnum"=w411) -> ("Avi Refnum (duplicate)"=w410:T6)  [unwired: 8 in, 1 out]
      }
    }
  }
  n170 = Close File(refnum=w27) -> ()  [unwired: 1 in, 2 out]
  n171 = case shown="True" w81 {
    tunnel: w83 -> [_ w423]
    frame False {
    }
    frame True {
      n172 = call "IMAQ AVI Close"("Avi Refnum"=w423) -> ()  [unwired: 10 in, 1 out]
    }
  }
  n173 = call <vilib>:"IMAQdx Close Camera.vi"("Session In"=w105) -> ("error out"=w106:errorcluster)  [unwired: 10 in]
  n174 = call "IMAQ Dispose"("Image"=w102) -> ()  [unwired: 5 in, 1 out]
  n175 = call <vilib>:"Simple Error Handler.vi"("error in (no error)"=w106) -> ()  [unwired: 4 in, 5 out]
